vi "I2C_WriteByteData.vi"(4 "Byte":u8 format="%.0x", 5 "Bus":i32=1, 6 "Device register":u8 format="%.0x", 7 "Address":u8 format="%.0x", 8 "error in":errorcluster) -> (0 "error out":errorcluster)   [LabVIEW 2014, in "GPIO.lvlib"]
doc: "Read a single byte from the specified I2C device"
uses:
  GPIO.lvlib
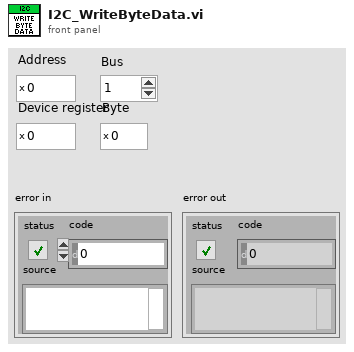
[diagram p1: front panel]
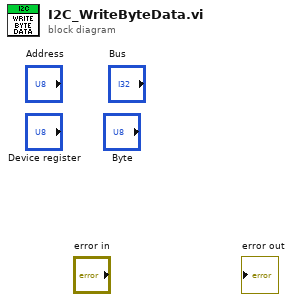
[diagram p0: block diagram]
diagram:
